vi "Set Sender.vi"(10 "Sender":refnum<class "Sender.lvclass">, 11 "TEMPLATE Msg Strategy in":refnum<class "TEMPLATE Msg Strategy.lvclass">) -> (3 "TEMPLATE Msg Strategy out":refnum<class "TEMPLATE Msg Strategy.lvclass">)   [LabVIEW 2021, in "_Template.lvlib" / "Templates.lvlib" / "TEMPLATE Msg Strategy.lvlib" / "TEMPLATE Msg Strategy.lvclass"]
uses:
  jettl/jettl/Sender/Sender/Sender.lvclass
  TEMPLATE Msg Strategy.lvclass
  TEMPLATE Msg Strategy.lvclass/TEMPLATE Msg Strategy.ctl
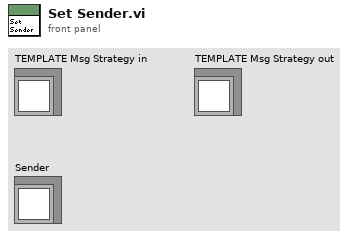
[diagram p1: front panel]
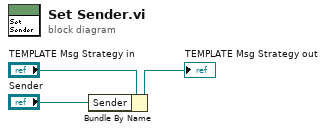
[diagram p0: block diagram]
diagram:
  n1 = Bundle By Name(cluster="TEMPLATE Msg Strategy in", "Sender"="Sender") -> (→"TEMPLATE Msg Strategy out":refnum<class "TEMPLATE Msg Strategy.lvclass">)
